vi "TLA_Execute Sql Query.vi"(8 "error in (no error)":errorcluster caption="错误输入（无错误）", 9 "SQLParam":refnum<k24>[](array[refnum]), 10 "SQLstring":string, 11 "Traceability 引用句柄":refnum<k24>) -> (0 "error out":errorcluster caption="错误输出", 1 "SQLParam 2":refnum<k24>[](array[refnum]), 2 ".NET:System.Data.DataTable":T1 {"RemotingFormat" items=["Xml", "Binary"]}, 3 "Traceability 引用句柄输出":refnum<k24>)   [LabVIEW 2014, in "Traceability.lvlib"]
uses:
  D:/webservice/Traceability.dll
  Traceability.dll
  System.Data
  Traceability.lvlib
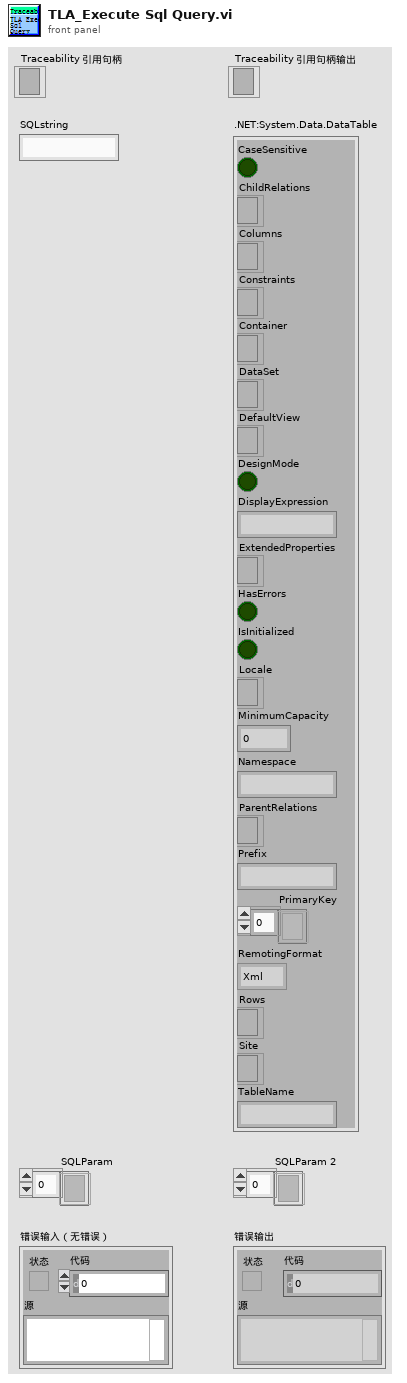
[diagram p1: front panel]
types:
  T1 = cluster{"CaseSensitive":bool, "ChildRelations":refnum<k24>, "Columns":refnum<k24>, "Constraints":refnum<k24>, "Container":refnum<k24>, "DataSet":refnum<k24>, "DefaultView":refnum<k24>, "DesignMode":bool, "DisplayExpression":string, "ExtendedProperties":refnum<k24>, "HasErrors":bool, "IsInitialized":bool, "Locale":refnum<k24>, "MinimumCapacity":i32, "Namespace":string, "ParentRelations":refnum<k24>, "Prefix":string, "PrimaryKey":refnum<k24>[], "RemotingFormat":i32, "Rows":refnum<k24>, "Site":refnum<k24>, "TableName":string}
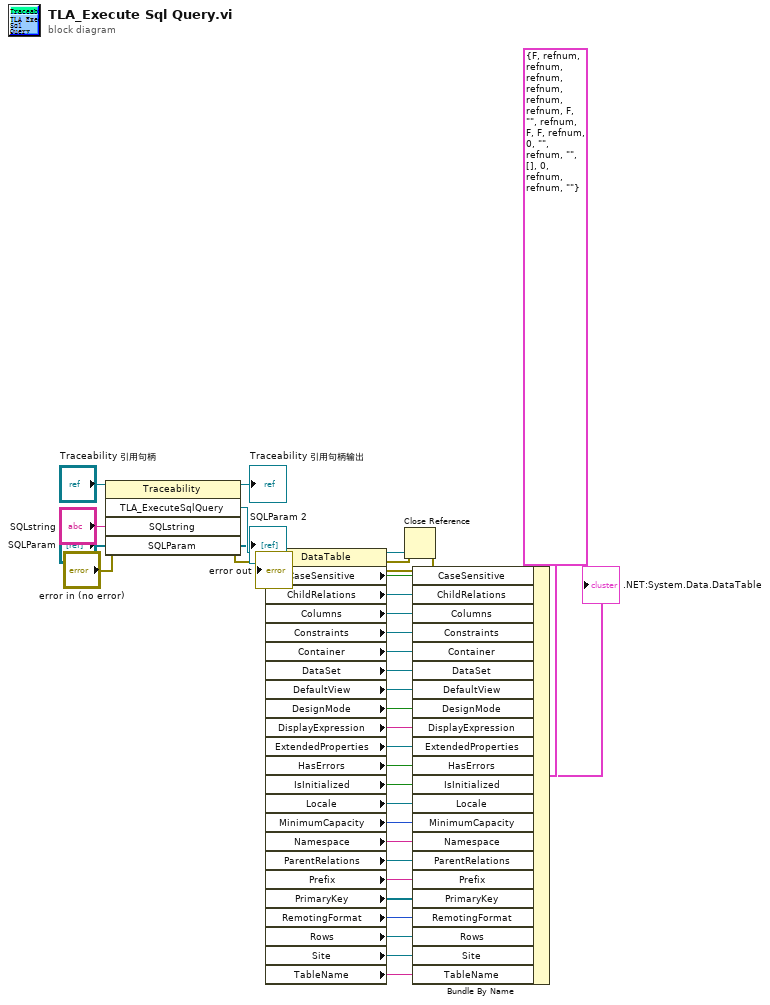
[diagram p0: block diagram]
diagram:
  n1 = invoke class="Traceability" method="TLA_ExecuteSqlQuery"(reference="Traceability 引用句柄", error in="error in (no error)", "SQLstring"="SQLstring", "SQLParam"="SQLParam") -> (reference out=→"Traceability 引用句柄输出":refnum<k24>, error out=w4:errorcluster, "TLA_ExecuteSqlQuery"=w32:refnum<k24>, "SQLParam"=→"SQLParam 2":refnum<k24>[])  [unwired: 1 in, 1 out]
  n2 = property class="DataTable"(reference=w32, error in=w4) -> (reference out=w3:refnum<k24>, error out=w2:errorcluster, "CaseSensitive"=w29:bool, "ChildRelations"=w28:refnum<k24>, "Columns"=w27:refnum<k24>, "Constraints"=w26:refnum<k24>, "Container"=w25:refnum<k24>, "DataSet"=w24:refnum<k24>, "DefaultView"=w23:refnum<k24>, "DesignMode"=w22:bool, "DisplayExpression"=w21:string, "ExtendedProperties"=w20:refnum<k24>, "HasErrors"=w19:bool, "IsInitialized"=w18:bool, "Locale"=w17:refnum<k24>, "MinimumCapacity"=w16:i32, "Namespace"=w15:string, "ParentRelations"=w14:refnum<k24>, "Prefix"=w13:string, "PrimaryKey"=w12:refnum<k24>[], "RemotingFormat"=w11:i32, "Rows"=w10:refnum<k24>, "Site"=w9:refnum<k24>, "TableName"=w8:string)
  n3 = Close Reference(reference=w3, error in (no error)=w2) -> (error out=→"error out":errorcluster)
  n4 = Bundle By Name(cluster=T1 {"CaseSensitive"=FALSE, "ChildRelations"=refnum, "Columns"=refnum, "Constraints"=refnum, "Container"=refnum, "DataSet"=refnum, "DefaultView"=refnum, "DesignMode"=FALSE, "DisplayExpression"="", "ExtendedProperties"=refnum, "HasErrors"=FALSE, "IsInitialized"=FALSE, "Locale"=refnum, "MinimumCapacity"=0, "Namespace"="", "ParentRelations"=refnum, "Prefix"="", "PrimaryKey"=[], "RemotingFormat"=0, "Rows"=refnum, "Site"=refnum, "TableName"=""} (".NET:System.Data.DataTable"), "CaseSensitive"=w29, "ChildRelations"=w28, "Columns"=w27, "Constraints"=w26, "Container"=w25, "DataSet"=w24, "DefaultView"=w23, "DesignMode"=w22, "DisplayExpression"=w21, "ExtendedProperties"=w20, "HasErrors"=w19, "IsInitialized"=w18, "Locale"=w17, "MinimumCapacity"=w16, "Namespace"=w15, "ParentRelations"=w14, "Prefix"=w13, "PrimaryKey"=w12, "RemotingFormat"=w11, "Rows"=w10, "Site"=w9, "TableName"=w8) -> (→".NET:System.Data.DataTable":T1)
